vi "Set IPS Switch Heater.vi"(8 "error in (no error)":errorcluster, 10 "Switch Heater Status":T1, 11 "Instrument.Oxford1820 in":refnum<class "Instrument.Oxford1820.lvclass">) -> (0 "error out":errorcluster, 2 "Response":string, 3 "Instrument.Oxford1820 out":refnum<class "Instrument.Oxford1820.lvclass">)   [LabVIEW 2016, in "Instrument.Oxford1820.lvclass"]
uses:
  Instrument.Oxford1820.lvclass
  <instrlib>/Mercury iXX/Public/Libraries/Magnet/Controls/Switch Heater.ctl
  Instrument.Oxford1820.lvclass/Instrument.Oxford1820.ctl
  <instrlib>/Mercury iXX/Public/Libraries/Magnet/Open/Open Magnet Device.vi
  <instrlib>/Mercury iXX/Public/Libraries/Magnet/Signals/Set/Switch Heater Status (Set).vi
  <instrlib>/Mercury iXX/Public/Libraries/Magnet/Signals/Read/Switch Heater Status (Read).vi
  <instrlib>/Mercury iXX/Mercury iXX.lvlib
  <instrlib>/Mercury iXX/Public/Libraries/Magnet.lvlib
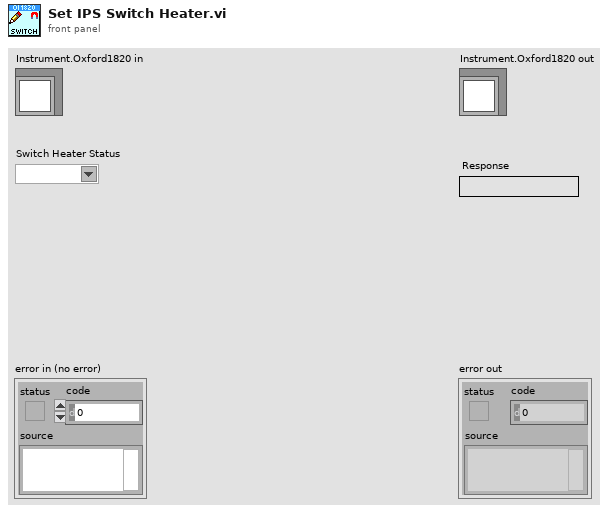
[diagram p1: front panel]
types:
  T1 = typedef "Mercury iXX.lvlib/Magnet.lvlib/Switch Heater.ctl" = string
  T2 = typedef "Mercury iXX.lvlib/Mercury Reference.ctl" = cluster{"Comms":refnum<visa-resource-name>, "Device ID":string[], "Comms Layer":T3, "Command":string, "Query reference":T4}
  T3 = typedef "Mercury iXX.lvlib/Comms Transport Layer.ctl" = enum16{"Ethernet TCP/IP", "USB", "ISOBus - RS-232", "GPIB"}
  T4 = typedef "Mercury iXX.lvlib/Query Dynamic Reference.ctl" = refnum<vi>
  T5 = typedef "Mercury iXX.lvlib/Response String.ctl" = string
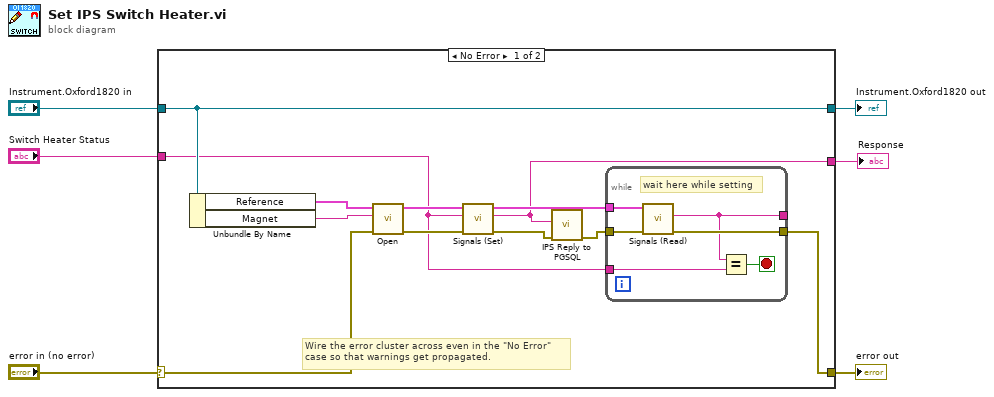
[diagram p0: block diagram]
diagram:
  n1 = case shown="No Error" "error in (no error)" {
    selector: "error in (no error)" -> [w15 w26]
    tunnel: [w8 w26] -> w5
    tunnel: [w18 w25] -> w3
    tunnel: "Instrument.Oxford1820 in" -> [w18 w25]
    tunnel: [w7 _] -> w2
    tunnel: "Switch Heater Status" -> [w10 _]
    frame No Error {
      # "Wire the error cluster across even in the \"No Error\"\ncase so that warnings get propagated."
      n2 = Unbundle By Name(w18) -> ("Reference"=w16:T2, "Magnet"=w17:string)
      n3 = call-poly <instrlib>:"Open.vi"("error in (no error)"=w15, "Device Identifier"=w17, "Mercury Reference In"=w16) -> ("error out"=w14:errorcluster, "Mercury Reference Out"=w13:T2)  [unwired: 7 out]
      n4 = call-poly <instrlib>:"Signals (Set).vi"("error in"=w14, "Switch Heater Status"=w10, "Mercury Reference In"=w13) -> ("error out"=w12:errorcluster, "Response"=w7:T5, "Mercury Reference Out"=w11:T2)  [unwired: 1 in, 5 out]
      n5 = call "IPS Reply to PGSQL.vi"("error in (no error)"=w12, "Response"=w7) -> ("error out"=w9:errorcluster)  [unwired: 9 in]
      n6 = while {
        tunnel: [w24] -> w8
        tunnel: w9 -> [w23]
        tunnel: w10 -> [w22]
        tunnel: w11 -> [w20]
        tunnel: [w19] -> _
        stop <- w21 stop-if-true
        # "wait here while setting"
        n7 = call-poly <instrlib>:"Signals (Read).vi"("error in"=w23, "Mercury Reference In"=w20) -> ("error out"=w24:errorcluster, "Switch Heater Status"=w19:string)  [unwired: 1 in, 7 out]
        n8 = Equal?(x=w19, y=w22) -> (x = y?=w21:bool)
      }
    }
    frame Error {
    }
  }
  "error out" <- w5
  "Instrument.Oxford1820 out" <- w3
  "Response" <- w2
